vi "QCP_Set.vi"   [LabVIEW 2016]
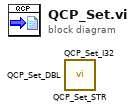
[diagram p0: block diagram]
diagram:
  n1 = call <userlib>:"QCP_Set_STR.vi"() -> ()  [unwired: 10 in, 1 out]
  n2 = call <userlib>:"QCP_Set_I32.vi"() -> ()  [unwired: 10 in, 1 out]
  n3 = call <userlib>:"QCP_Set_DBL.vi"() -> ()  [unwired: 10 in, 1 out]
